vi "Timer Update Display.vi"(8 "error in (no error)":errorcluster, 9 "Current Time":dbl, 10 "Starting Time":dbl, 11 "Controller in":refnum<class "Controller.lvclass">) -> (0 "error out":errorcluster, 3 "Controller out":refnum<class "Controller.lvclass">)   [LabVIEW 2021, in "Controller.lvlib" / "Controller.lvclass"]
uses:
  Controller.lvclass
  Controller.lvclass/Controller.ctl
  MC Prompt/MC Prompt Messages/Update Timer Display Msg/Update Timer Display Msg.lvclass/Update Timer Display Msg.ctl
  <vilib>/ActorFramework/Message Enqueuer/Message Enqueuer.lvclass/Message Enqueuer.ctl
  <vilib>/ActorFramework/Message Enqueuer/Enqueue.vi
  MC Prompt/MC Prompt Messages/Update Timer Display Msg/Update Timer Display Msg.lvclass
  C:/Program Files/National Instruments/LabVIEW 2024/vi.lib/ActorFramework/Message/Message.lvclass
  <vilib>/ActorFramework/Message Priority Queue/Priority Enqueue.vi
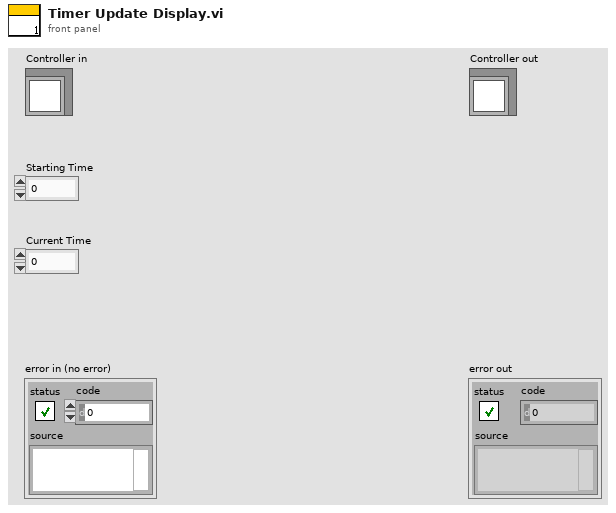
[diagram p1: front panel]
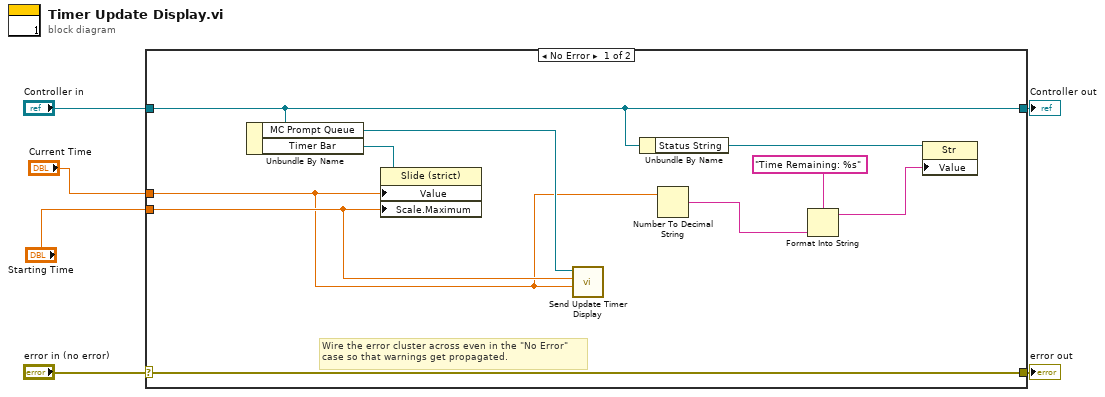
[diagram p0: block diagram]
diagram:
  n1 = case shown="No Error" "error in (no error)" {
    selector: "error in (no error)" -> [w16 w18]
    tunnel: [w16 w18] -> w5
    tunnel: [w13 w17] -> w3
    tunnel: "Controller in" -> [w13 w17]
    tunnel: "Starting Time" -> [w12 _]
    tunnel: "Current Time" -> [w10 _]
    frame No Error {
      # "Wire the error cluster across even in the \"No Error\"\ncase so that warnings get propagated."
      n2 = Unbundle By Name(w13) -> ("MC Prompt Queue"=w14:refnum<class "Message Enqueuer.lvclass">, "Timer Bar"=w15:refnum<vi>)
      n3 = property class="Slide (strict)"(reference=w15, "Value"=w10, "Scale.Maximum"=w12) -> ()  [unwired: 1 in, 2 out]
      n4 = call "Send Update Timer Display.vi"("Current Time"=w10, "Starting Time"=w12, "Message Enqueuer"=w14) -> ()  [unwired: 7 in, 2 out]
      n5 = Unbundle By Name(w13) -> ("Status String"=w11:refnum<vi>)
      n6 = Number To Decimal String(number=w10) -> (decimal integer string=w8:string)  [unwired: 1 in]
      n7 = Format Into String(format string="Time Remaining: %s", w8) -> (resulting string=w7:string)  [unwired: 2 in, 1 out]
      n8 = property class="Str"(reference=w11, "Value"=w7) -> ()  [unwired: 1 in, 2 out]
    }
    frame Error {
    }
  }
  "error out" <- w5
  "Controller out" <- w3
